vi "Configure Correction.vi"(0 "VISA resource name":refnum<visa-resource-name>, 1 "Enable Correction (T: Enable)":bool=TRUE, 2 "Frequency Array":dbl[](array[numeric])=[27000000000.0, 27000000000.0], 3 "Amplitude Array":dbl[](array[numeric])=[0.0, 0.0], 5 "Correction Set (1: Antenna)":u16(ring)=1 items=["Antenna"=1, "Cable"=2, "Other"=3, "User"=4], 7 "Frequency Interpolation (0: Linear)":u16(ring) items=["Linear", "Logarithmic"], 11 "error in (no error)":errorcluster) -> (4 "VISA resource name out":refnum<visa-resource-name>, 15 "error out":errorcluster)   [LabVIEW 2014, in "Agilent ESA PSA Series.lvlib"]
doc: "Configures Correction."
uses:
  Agilent ESA PSA Series.lvlib
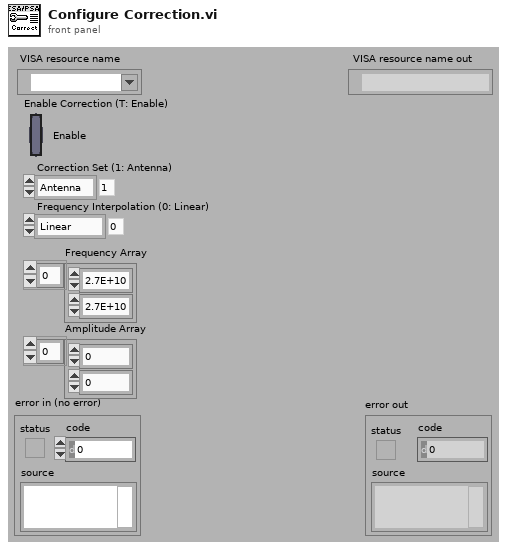
[diagram p1: front panel]
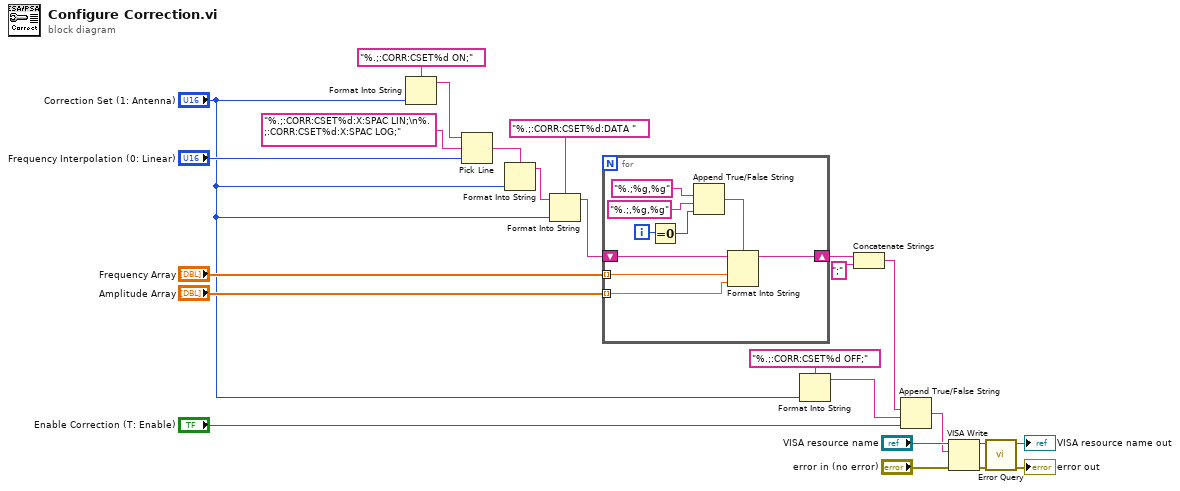
[diagram p0: block diagram]
diagram:
  n1 = Format Into String(format string="%.;:CORR:CSET%d ON;", "Correction Set (1: Antenna)") -> (resulting string=w6:string)  [unwired: 2 in, 1 out]
  n2 = Pick Line(string ("")=w6, multi-line string="%.;:CORR:CSET%d:X:SPAC LIN;\n%.;:CORR:CSET%d:X:SPAC LOG;" ("string (\"\")"), line index="Frequency Interpolation (0: Linear)") -> (output string=w13:string)
  n3 = Format Into String(format string=w13, "Correction Set (1: Antenna)") -> (resulting string=w8:string)  [unwired: 2 in, 1 out]
  n4 = Format Into String(format string="%.;:CORR:CSET%d:DATA ", initial string=w8, "Correction Set (1: Antenna)") -> (resulting string=w10:string)  [unwired: 1 in, 1 out]
  n5 = for {
    tunnel: "Frequency Array" -> [w28] mode=indexing
    shift-right: [w27] -> w4
    shift-left: w10 -> [w26]
    tunnel: "Amplitude Array" -> [w25] mode=indexing
    i -> [w33]
    n6 = Equal To 0?(x=w33) -> (x = 0?=w32:bool)
    n7 = Append True/False String(1:w32, 2:"%.;,%g,%g" ("format string"), 3:"%.;%g,%g" ("format string")) -> (0:w29:string)  [unwired: 1 in]
    n8 = Format Into String(format string=w29, initial string=w26, w28, w25) -> (resulting string=w27:string)  [unwired: 1 in, 1 out]
  }
  n9 = Format Into String(format string="%.;:CORR:CSET%d OFF;", "Correction Set (1: Antenna)") -> (resulting string=w16:string)  [unwired: 2 in, 1 out]
  n10 = Concatenate Strings(w4, ";" ("string")) -> (w2:string)
  n11 = Append True/False String(1:"Enable Correction (T: Enable)", 2:w16, 3:w2) -> (0:w5:string)  [unwired: 1 in]
  n12 = VISA Write(VISA resource name="VISA resource name", write buffer=w5, error in (no error)="error in (no error)") -> (VISA resource name out=w22:refnum<visa-resource-name>, error out=w20:errorcluster)  [unwired: 1 out]
  n13 = call "Error Query.vi"("error in (no error)"=w20, "VISA resource name"=w22) -> ("error out"=→"error out":errorcluster, "VISA resource name out"=→"VISA resource name out":refnum<visa-resource-name>)  [unwired: 6 in, 2 out]
